vi "Configure SMU Negative Current Limit.vi"(8 "error in (no error)":errorcluster {"code" format="%.0x"}, 9 "Negative Current Limit (0.0 amps)":dbl format="%^.3e", 10 "Channel Name (1)":string="1", 11 "VISA resource name":refnum<visa-resource-name>) -> (0 "error out":errorcluster {"code" format="%.0x"}, 3 "VISA resource name out":refnum<visa-resource-name>)   [LabVIEW 2014, in "Agilent N6700 Series.lvlib"]
doc: "Sets the negative current limit of the specified output channel.\n\n<b>Notes:</b>\n(1) The output protection priority must be set to voltage in <b>Configure Output Regulation.vi</b>.\n(2) This VI only applies to N678xA SMU and N6783A-BAT."
uses:
  Agilent N6700 Series.lvlib
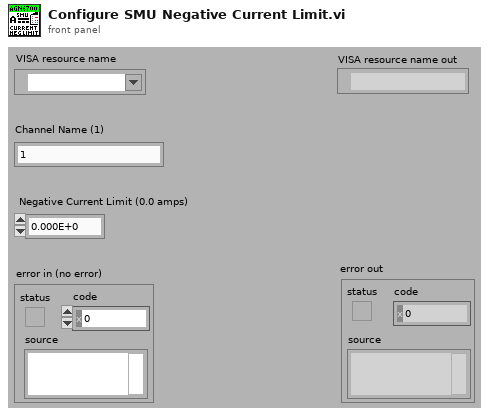
[diagram p1: front panel]
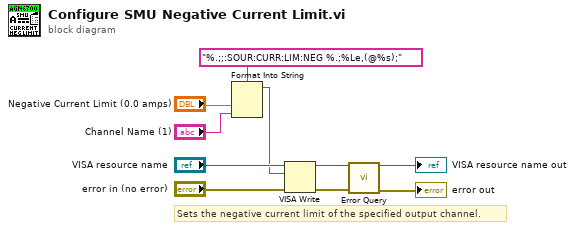
[diagram p0: block diagram]
diagram:
  # "Sets the negative current limit of the specified output channel."
  n1 = Format Into String(format string="%.;;:SOUR:CURR:LIM:NEG %.;%Le,(@%s);", "Negative Current Limit (0.0 amps)", "Channel Name (1)") -> (resulting string=w4:string)  [unwired: 2 in, 1 out]
  n2 = VISA Write(VISA resource name="VISA resource name", write buffer=w4, error in (no error)="error in (no error)") -> (VISA resource name out=w6:refnum<visa-resource-name>, error out=w5:errorcluster)  [unwired: 1 out]
  n3 = call "Error Query.vi"("VISA resource name"=w6, "error in (no error)"=w5) -> ("VISA resource name out"=→"VISA resource name out":refnum<visa-resource-name>, "error out"=→"error out":errorcluster)  [unwired: 10 in, 2 out]
